vi "_ConnectorPaneEditor_AllowEditCell.vi"(8 "error in (no error)":errorcluster, 10 "Cell Position":T1, 11 "ConnectorPaneEditor in":refnum<class "_ConnectorPaneEditor.lvclass">) -> (0 "error out":errorcluster, 1 "EditPos":T1, 2 "Allow?":bool, 3 "ConnectorPaneEditor out":refnum<class "_ConnectorPaneEditor.lvclass">)   [LabVIEW 2014, in "_ConnectorPaneEditor.lvclass"]
uses:
  _ConnectorPaneEditor.lvclass
  <vilib>/Utility/miscctls.llb/LVRowAndColumnTypeDef.ctl
  _ConnectorPaneEditor.lvclass/_ConnectorPaneEditor.ctl
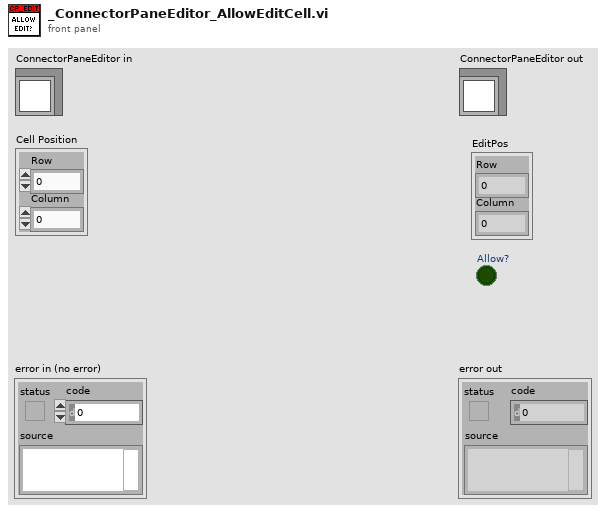
[diagram p1: front panel]
types:
  T1 = typedef "LVRowAndColumnTypeDef.ctl" = cluster{"Row":i32, "Column":i32}
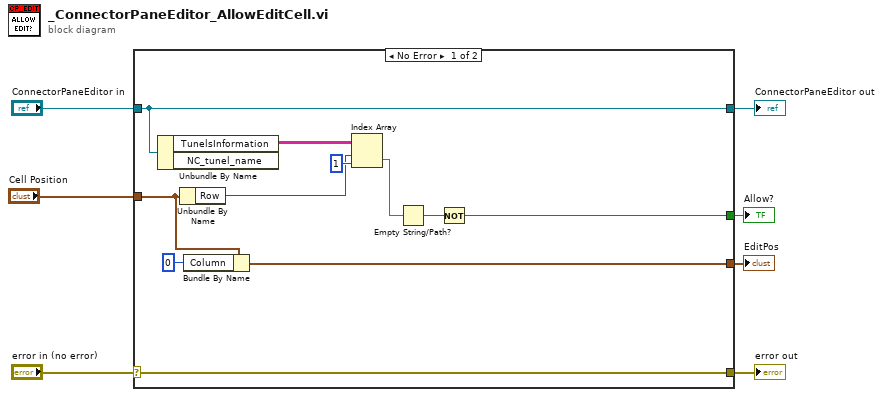
[diagram p0: block diagram]
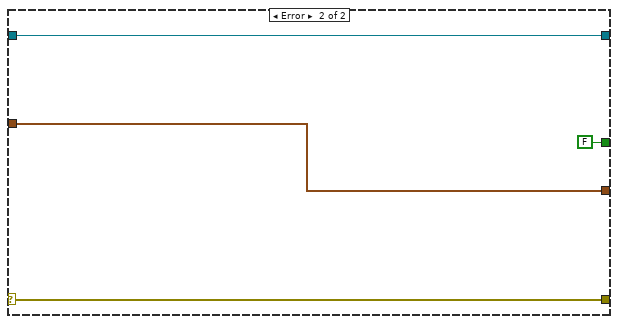
[diagram p2: hidden frame]
diagram:
  n1 = case shown="No Error" "error in (no error)" {
    selector: "error in (no error)" -> [w18 w22]
    tunnel: [w18 w22] -> w6
    tunnel: [w17 w21] -> w4
    tunnel: "ConnectorPaneEditor in" -> [w17 w21]
    tunnel: "Cell Position" -> [w13 w19]
    tunnel: [w11 w19] -> w2
    tunnel: [w8 FALSE] -> w1
    frame No Error {
      n2 = Unbundle By Name(w17) -> ("TunelsInformation"=w16:string[][])  [unwired: 1 out]
      n3 = Unbundle By Name(w13) -> ("Row"=w14:i32)
      n4 = Bundle By Name(cluster=w13, "Column"=0) -> (w11:T1)
      n5 = Index Array(array=w16, index (row)=w14, index (col)=1 ("disabled index (col)")) -> (element=w10:string)
      n6 = Empty String/Path?(string/path=w10) -> (empty?=w9:bool)
      n7 = Not(x=w9) -> (.not. x?=w8:bool)
    }
    frame Error {
    }
  }
  "error out" <- w6
  "ConnectorPaneEditor out" <- w4
  "EditPos" <- w2
  "Allow?" <- w1
